vi "Send Request (Async).vi"(8 "error in (no error)":errorcluster, 10 "JSON Request String":string, 11 "Server in":refnum<class "JSONRPC Server.lvclass">) -> (0 "error out":errorcluster, 1 "notification?":bool, 2 "id value":string, 3 "Server out":refnum<class "JSONRPC Server.lvclass">)   [LabVIEW 2015, in "JSONRPC Server.lvclass"]
uses:
  JSONRPC Server.lvclass
  Request/Request.lvclass
  Request/Request.lvclass/Request.ctl
  Request/Read id value.vi
  id/id.lvclass
  JSONable/JSONable.lvclass
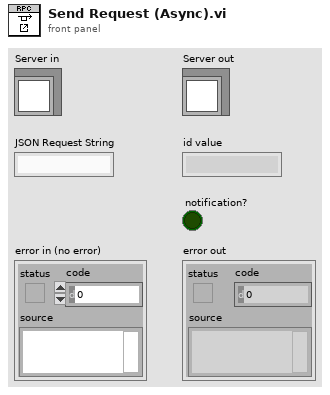
[diagram p1: front panel]
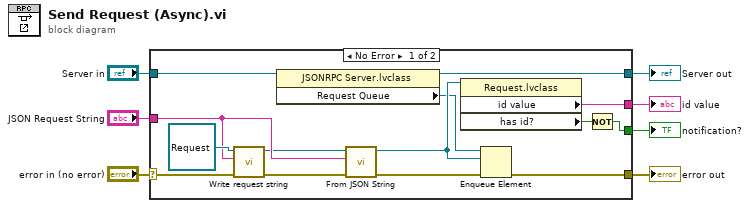
[diagram p0: block diagram]
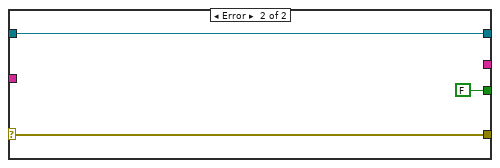
[diagram p2: hidden frame]
diagram:
  n1 = case shown="No Error" "error in (no error)" {
    selector: "error in (no error)" -> [w12 w24]
    tunnel: [w20 w24] -> w6
    tunnel: [w8 w23] -> w4
    tunnel: "Server in" -> [w10 w23]
    tunnel: "JSON Request String" -> [w14 _]
    tunnel: [w18 _] -> w2
    tunnel: [w16 FALSE] -> w1
    frame No Error {
      n2 = call "Write request string.vi"("error in (no error)"=w12, "request string"=w14, "Request in"=refnum<class "Request.lvclass"> refnum ("Request.lvclass")) -> ("error out"=w11:errorcluster, "Request out"=w13:refnum<class "Request.lvclass">)  [unwired: 7 in]
      n3 = property class="JSONRPC Server.lvclass"(reference=w10) -> (reference out=w8:refnum<class "JSONRPC Server.lvclass">, "Request Queue"=w9:refnum<queue>)  [unwired: 1 in, 1 out]
      n4 = call "From JSON String.vi"("error in (no error)"=w11, "JSON String"=w14, "JSONable in"=w13) -> ("error out"=w21:errorcluster, "JSONable out"=w19:refnum<class "Request.lvclass">)  [unwired: 7 in]
      n5 = property class="Request.lvclass"(reference=w19) -> ("id value"=w18:string, "has id?"=w17:bool)  [unwired: 1 in, 2 out]
      n6 = Enqueue Element(queue=w9, element=w19, error in (no error)=w21) -> (error out=w20:errorcluster)  [unwired: 1 in, 2 out]
      n7 = Not(x=w17) -> (.not. x?=w16:bool)
    }
    frame Error {
    }
  }
  "error out" <- w6
  "Server out" <- w4
  "id value" <- w2
  "notification?" <- w1
